vi "Periodic Tasks.vi"(8 "error in":errorcluster) -> ()   [LabVIEW 2017]
doc: "This VI runs in parallel to other tasks. It can contain as many user-defined periodic loops as you need. These can carry out PID or other sorts of timed response."
uses:
  <vilib>/Rock Robotics/WPI/Utilities/WPI_GetSetVariantRefNum.vi
  Robot Global Data.vi
  <vilib>/Rock Robotics/Network Tables/NT Write Number.vi
  <vilib>/Rock Robotics/WPI/ThirdParty/Phoenix-LabVIEW/Motor Controller/Get/CTRE_Phoenix_MotorController_GetOutputCurrent_Enhanced.vi
  <vilib>/Rock Robotics/WPI/ThirdParty/Phoenix-LabVIEW/Motor Controller/Get/CTRE_Phoenix_MotorController_GetQuadratureData.vi
panel:
  out "ARM 3 FEEDBACK":dbl
  out "ARM 2 FEEDBACK":dbl
  out "ARM 1 FEEDBACK":dbl
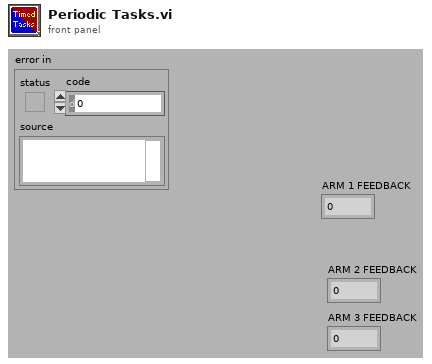
[diagram p1: front panel]
types:
  T1 = typedef "WPI_JoystickDevRef.ctl" = cluster{"Device":T2}
  T2 = typedef "WPI_JoystickDeviceEnum.ctl" = enum16{"USB 0", "USB 1", "USB 2", "USB 3", "USB 4", "USB 5"}
  T3 = typedef "WPI_RobotDriveDevRef.ctl" = cluster{"DevStatus":errorcluster, "Motors[]":T4[], "Square Inputs":bool, "Max Output":dbl}
  T4 = typedef "WPI_MotorControlDeviceRef.ctl" = cluster{"DeviceStatus":errorcluster, "Type":T5, "PWM":cluster{"PWM Channel":T6, "DeadBand":T7}, "CAN":cluster{"Device Number":u8, "SetOutput VI Ref":variant, "GetOutput VI Ref":variant, "Enable VI Ref":variant, "Disable VI Ref":variant, "Data":variant}, "Invert":bool, "DIO PWM":cluster{"PWM \"Enable\" Channel":T6, "DIOChannel":T8, "PWM Rate":dbl}}
  T5 = typedef "WPI_MotorControlType.ctl" = enum16{"PWM", "CAN", "DIO PWM"}
  T6 = typedef "FPGA_DIOPWMChannel.ctl" = enum8{"PWM 0", "PWM 1", "PWM 2", "PWM 3", "PWM 4", "PWM 5", "PWM 6", "PWM 7", "PWM 8", "PWM 9", "PWM MXP 0", "PWM MXP 1", "PWM MXP 2", "PWM MXP 3", "PWM MXP 4", "PWM MXP 5", "PWM MXP 6", "PWM MXP 7", "PWM MXP 8", "PWM MXP 9", "Invalid"}
  T7 = typedef "WPI_PWMDeadband.ctl" = cluster{"Name":string, "maxPositivePwm":i32, "minPositivePwm":i32, "centerPwm":i32, "maxNegativePwm":i32, "minNegativePwm":i32, "angularRange":u16}
  T8 = typedef "FPGA_DIOChannel.ctl" = enum8{"DIO 0", "DIO 1", "DIO 2", "DIO 3", "DIO 4", "DIO 5", "DIO 6", "DIO 7", "DIO 8", "DIO 9", "DIO MXP 0", "DIO MXP 1", "DIO MXP 2", "DIO MXP 3", "DIO MXP 4", "DIO MXP 5", "DIO MXP 6", "DIO MXP 7", "DIO MXP 8", "DIO MXP 9", "DIO MXP 10", "DIO MXP 11", "DIO MXP 12", "DIO MXP 13", "DIO MXP 14", "DIO MXP 15", "SPI Port CS1", "SPI Port CS2", "SPI Port CS3", "SPI Port MISO", "SPI Port MOSI", "Invalid"}
  T9 = cluster{"JoystickDevRef":T1, "RobotDriveDevRef":T3}
  T10 = cluster{"Yaw":dbl, "Roll":dbl, "Pitch":dbl, "Heading":dbl, "Fused Heading":dbl}
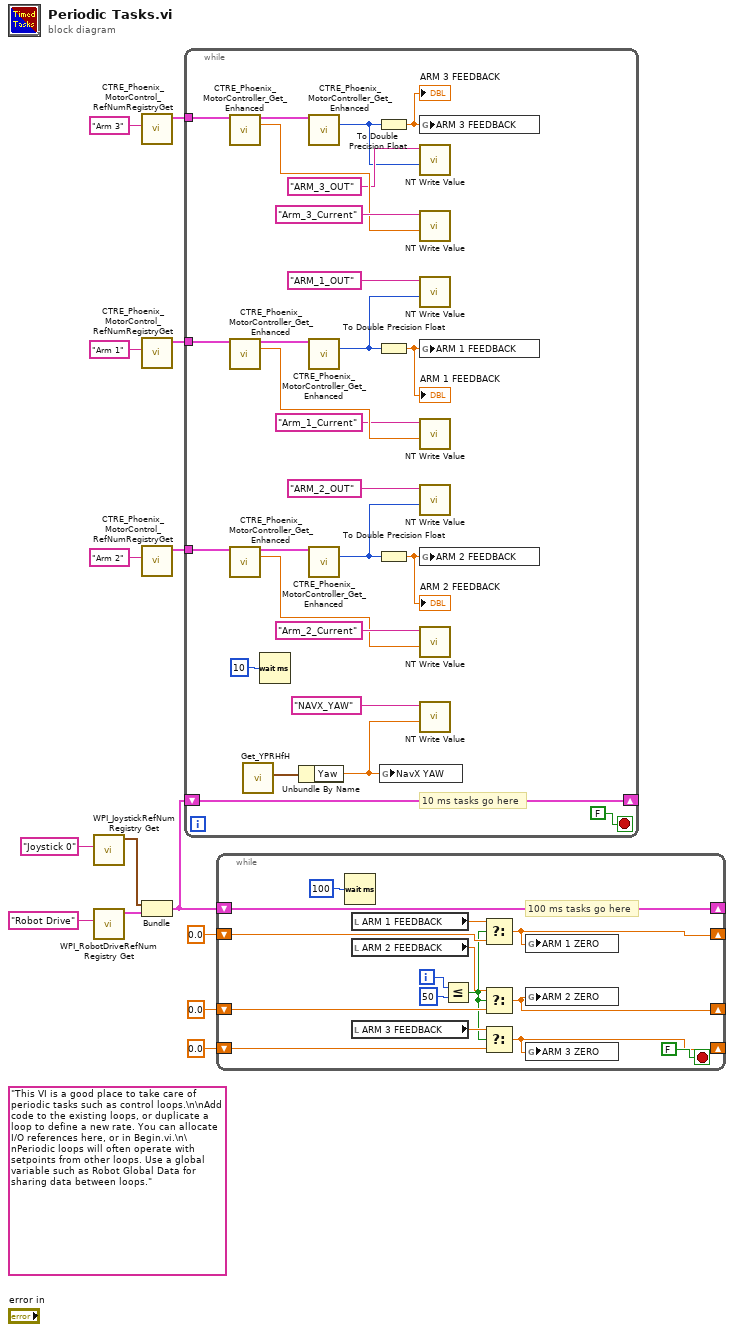
[diagram p0: block diagram]
diagram:
  (unwired) "This VI is a good place to take care of periodic tasks such as control loops.\n\nAdd code to the existing loops, or duplicate a loop to define a new rate. You can allocate I/O references here, or in Begin.vi.\n\nPeriodic loops will often operate with setpoints from other loops. Use a global variable such as Robot Global Data for sharing data between loops."
  n1 = call <vilib>:"WPI_JoystickRefNum Registry Get.vi"("refnum name"="Joystick 0") -> ("JoystickDevRef"=w12:T1)  [unwired: 1 in, 9 out]
  n2 = call <vilib>:"WPI_RobotDriveRefNum Registry Get.vi"("refnum name"="Robot Drive") -> ("RobotDriveDevRef"=w11:T3)  [unwired: 1 in, 9 out]
  n3 = call <vilib>:"CTRE_Phoenix_MotorControl_RefNumRegistryGet.vi"("refnum name"="Arm 3") -> ("PhoenixMotorControlDevRef"=w5:T4)  [unwired: 9 in, 1 out]
  n4 = call <vilib>:"CTRE_Phoenix_MotorControl_RefNumRegistryGet.vi"("refnum name"="Arm 1") -> ("PhoenixMotorControlDevRef"=w6:T4)  [unwired: 9 in, 1 out]
  n5 = call <vilib>:"CTRE_Phoenix_MotorControl_RefNumRegistryGet.vi"("refnum name"="Arm 2") -> ("PhoenixMotorControlDevRef"=w4:T4)  [unwired: 9 in, 1 out]
  n6 = Bundle("JoystickDevRef"=w12, "RobotDriveDevRef"=w11) -> (w10:T9)  [unwired: 1 out]
  n7 = while {
    shift-right: [w27] -> _
    shift-left: w10 -> [w27]
    tunnel: w6 -> [w39]
    tunnel: w5 -> [w38]
    tunnel: w4 -> [w37]
    stop <- FALSE stop-if-true
    # "10 ms tasks go here"
    n8 = call-poly <vilib>:"CTRE_Phoenix_MotorController_Get_Enhanced.vi"("PhoenixMotorControlDevRef"=w38) -> ("PhoenixMotorControlDevRef"=w28:T4, "Output Current"=w32:dbl)  [unwired: 12 in, 1 out]
    n9 = call-poly <vilib>:"CTRE_Phoenix_MotorController_Get_Enhanced.vi"("PhoenixMotorControlDevRef"=w39) -> ("PhoenixMotorControlDevRef"=w30:T4, "Output Current"=w36:dbl)  [unwired: 12 in, 1 out]
    n10 = call-poly <vilib>:"CTRE_Phoenix_MotorController_Get_Enhanced.vi"("PhoenixMotorControlDevRef"=w37) -> ("PhoenixMotorControlDevRef"=w29:T4, "Output Current"=w31:dbl)  [unwired: 12 in, 1 out]
    n11 = call <vilib>:"Get_YPRHfH.vi"() -> ("YRPHfH"=w20:T10)  [unwired: 11 in]
    n12 = Wait (ms)(milliseconds to wait=u32 10) -> ()  [unwired: 1 out]
    n13 = Unbundle By Name(w20) -> ("Yaw"=w18:dbl)
    n14 = call-poly <vilib>:"CTRE_Phoenix_MotorController_Get_Enhanced.vi"("PhoenixMotorControlDevRef"=w28) -> ("Quadrature Position"=w21:i32)  [unwired: 11 in, 3 out]
    n15 = call-poly <vilib>:"CTRE_Phoenix_MotorController_Get_Enhanced.vi"("PhoenixMotorControlDevRef"=w30) -> ("Quadrature Position"=w23:i32)  [unwired: 11 in, 3 out]
    n16 = call-poly <vilib>:"CTRE_Phoenix_MotorController_Get_Enhanced.vi"("PhoenixMotorControlDevRef"=w29) -> ("Quadrature Position"=w22:i32)  [unwired: 11 in, 3 out]
    n17 = To Double Precision Float(number=w21) -> (double precision float=w15:dbl)
    "ARM 3 FEEDBACK" <- w15
    n18 = To Double Precision Float(number=w23) -> (double precision float=w17:dbl)
    "ARM 1 FEEDBACK" <- w17
    n19 = To Double Precision Float(number=w22) -> (double precision float=w16:dbl)
    "ARM 2 FEEDBACK" <- w16
    n20 = global write "Robot Global Data.vi" "NavX YAW"(w18) -> ()
    n21 = global write "Robot Global Data.vi" "ARM 3 FEEDBACK"(w15) -> ()
    n22 = call-poly <vilib>:"NT Write Value.vi"("Numeric"=w21, "Name"="ARM_3_OUT") -> ()  [unwired: 9 in, 1 out]
    n23 = call-poly <vilib>:"NT Write Value.vi"("Numeric"=w32, "Name"="Arm_3_Current") -> ()  [unwired: 9 in, 1 out]
    n24 = call-poly <vilib>:"NT Write Value.vi"("Numeric"=w23, "Name"="ARM_1_OUT") -> ()  [unwired: 9 in, 1 out]
    n25 = global write "Robot Global Data.vi" "ARM 1 FEEDBACK"(w17) -> ()
    n26 = call-poly <vilib>:"NT Write Value.vi"("Numeric"=w36, "Name"="Arm_1_Current") -> ()  [unwired: 9 in, 1 out]
    n27 = call-poly <vilib>:"NT Write Value.vi"("Numeric"=w22, "Name"="ARM_2_OUT") -> ()  [unwired: 9 in, 1 out]
    n28 = global write "Robot Global Data.vi" "ARM 2 FEEDBACK"(w16) -> ()
    n29 = call-poly <vilib>:"NT Write Value.vi"("Numeric"=w31, "Name"="Arm_2_Current") -> ()  [unwired: 9 in, 1 out]
    n30 = call-poly <vilib>:"NT Write Value.vi"("Numeric"=w18, "Name"="NAVX_YAW") -> ()  [unwired: 9 in, 1 out]
  }
  n31 = while {
    shift-right: [w54] -> _
    shift-left: w10 -> [w54]
    shift-right: [w52] -> _
    shift-left: 0.0 ("ARM 1 FEEDBACK") -> [w51]
    shift-right: [w49] -> _
    shift-left: 0.0 ("ARM 2 FEEDBACK") -> [w48]
    shift-right: [w45] -> _
    shift-left: 0.0 ("ARM 2 FEEDBACK") -> [w46]
    i -> [w43]
    stop <- FALSE stop-if-true
    # "100 ms tasks go here"
    n32 = Wait (ms)(milliseconds to wait=u32 100) -> ()  [unwired: 1 out]
    n33 = local read "ARM 1 FEEDBACK"() -> (w53:dbl)
    n34 = local read "ARM 2 FEEDBACK"() -> (w50:dbl)
    n35 = local read "ARM 3 FEEDBACK"() -> (w47:dbl)
    n36 = Less Or Equal?(x=w43, y=50) -> (x <= y?=w42:bool)
    n37 = Select(t=w53, s=w42, f=w51) -> (s? t:f=w52:dbl)
    n38 = Select(t=w50, s=w42, f=w48) -> (s? t:f=w49:dbl)
    n39 = Select(t=w47, s=w42, f=w46) -> (s? t:f=w45:dbl)
    n40 = global write "Robot Global Data.vi" "ARM 1 ZERO"(w52) -> ()
    n41 = global write "Robot Global Data.vi" "ARM 2 ZERO"(w49) -> ()
    n42 = global write "Robot Global Data.vi" "ARM 3 ZERO"(w45) -> ()
  }
